vi "Make Array.vi"(3 "Error In":errorcluster, 4 "Step":dbl=0.01, 5 "New":dbl, 6 "Old":dbl) -> (0 "Error Out":errorcluster, 1 "Array":dbl[](array[numeric]), 2 "Samples":i32)   [LabVIEW 2012]
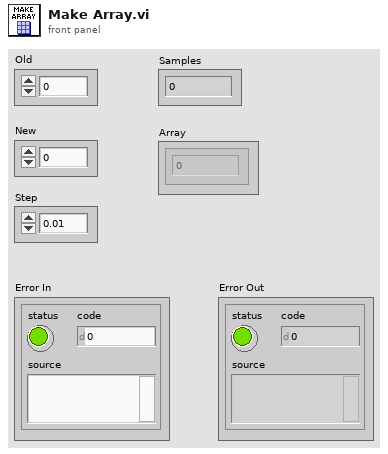
[diagram p1: front panel]
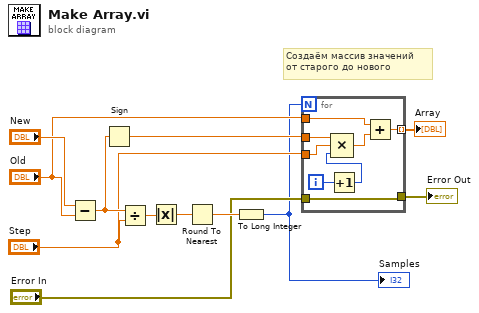
[diagram p0: block diagram]
diagram:
  # "Создаём массив значений\nот старого до нового"
  n1 = Subtract(x="New", y="Old") -> (x-y=w7:dbl)
  n2 = Sign(1:w7) -> (0:w6:dbl)
  n3 = Divide(x=w7, y="Step") -> (x/y=w9:dbl)
  n4 = Absolute Value(x=w9) -> (abs(x)=w8:dbl)
  n5 = Round To Nearest(number=w8) -> (nearest integer value=w12:dbl)
  n6 = To Long Integer(number=w12) -> (32bit integer=w1:i32)
  "Samples" <- w1
  n7 = for {
    N: w1 -> [_]
    tunnel: "Old" -> [w19]
    tunnel: [w18] -> w5 mode=indexing
    tunnel: "Step" -> [w15]
    tunnel: w6 -> [w17]
    tunnel: "Error In" -> [w13]
    tunnel: [w13] -> w3
    i -> [w20]
    n8 = Increment(x=w20) -> (x+1=w14:i32)
    n9 = Compound Arithmetic op=MULTIPLY(w17, w15, w14) -> (w16:dbl)
    n10 = Add(x=w19, y=w16) -> (x+y=w18:dbl)
  }
  "Array" <- w5
  "Error Out" <- w3
